vi "TakeAction.vi"(0 "Account Info":T1, 5 "Action":string, 7 "User input":string, 9 "Array":refnum<vi>[](array[refnum]), 11 "Error in":errorcluster) -> (4 "Get Message":string, 6 "Left menu":cluster{"L1":string, "L2":string, "L3":string}, 8 "Right Menu":cluster{"R1":string, "R2":string, "R3":string}, 10 "Updated acc info":T1, 15 "Error out":errorcluster)   [LabVIEW 2017]
doc: "This VI takes the appropriate action based on the action performed on the front panel. It also provides the output based on the action"
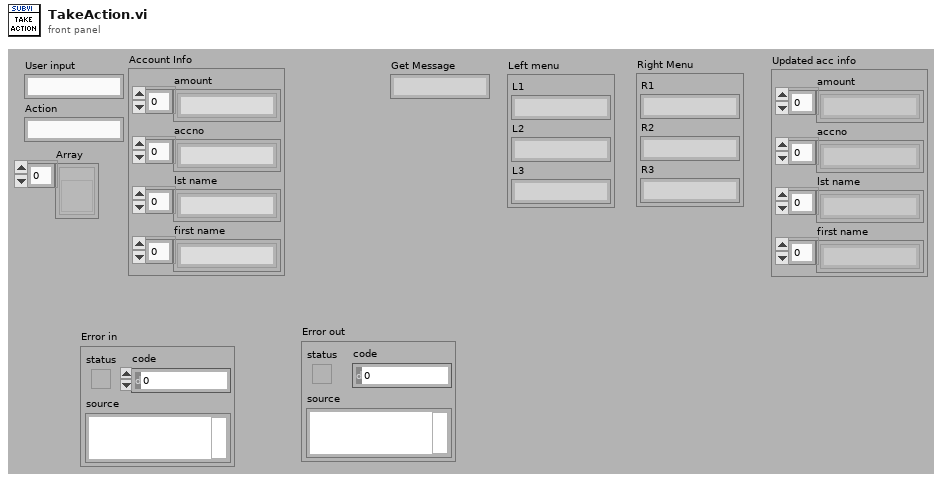
[diagram p1: front panel]
types:
  T1 = cluster{"amount":string[], "accno":string[], "lst name":string[], "first name":string[]}
  T2 = enum8{"Enabled", "Disabled", "Disabled and Grayed Out"}
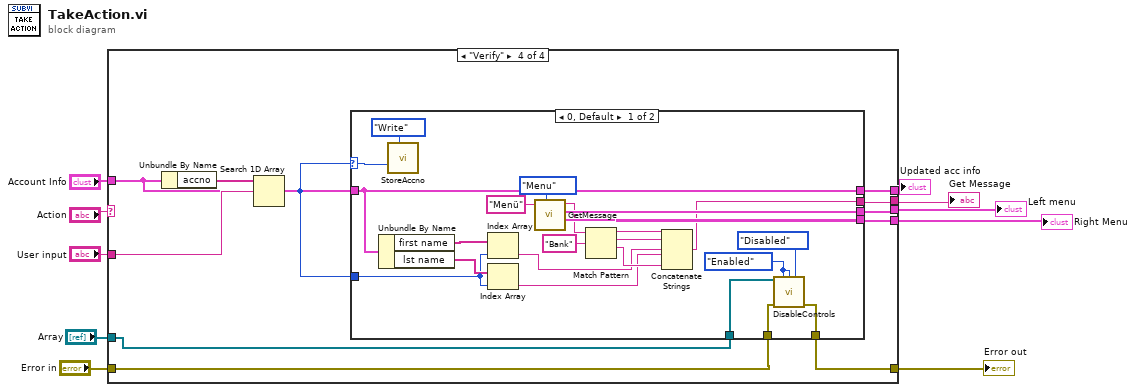
[diagram p0: block diagram]
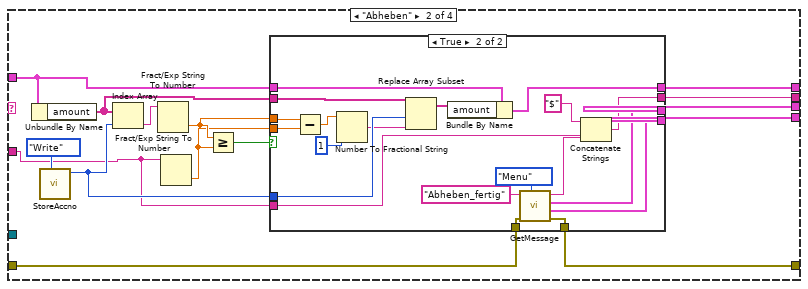
[diagram p3: hidden frame]
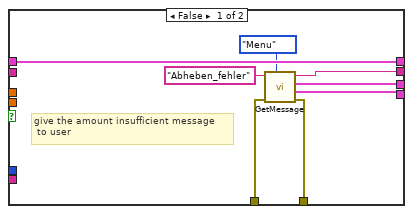
[diagram p4: hidden frame]
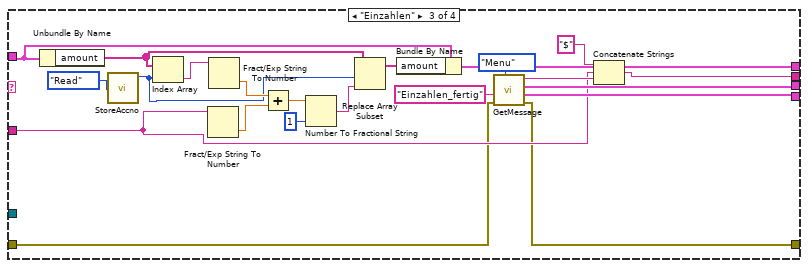
[diagram p5: hidden frame]
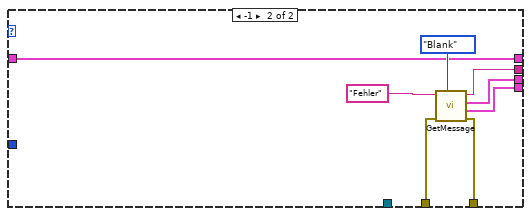
[diagram p6: hidden frame]
diagram:
  n1 = case shown="\"Verify\"" "Action" {
    tunnel: "User input" -> [_ w15 w58 w87]
    tunnel: "Account Info" -> [w12 w20 w73 w83]
    tunnel: [_ w16 w60 w86] -> w7
    tunnel: [_ w18 w66 w85] -> w6
    tunnel: [_ w17 w65 w84] -> w5
    tunnel: [w12 w19 w68 w82] -> w4
    tunnel: "Array" -> [_ _ _ w80]
    tunnel: "Error in" -> [w11 w14 w57 w79]
    tunnel: [w11 w13 w56 w78] -> w1
    frame Default {
    }
    frame "Abheben" {
      n2 = Unbundle By Name(w20) -> ("amount"=w21:string[])
      n3 = call "StoreAccno.vi"("Enum"=enum16{"Read", "Write"}."Write") -> ("Read"=w22:i32)  [unwired: 10 in]
      n4 = Index Array(array=w21, index=w22) -> (element=w26:string)
      n5 = Fract/Exp String To Number(string=w26) -> (number=w24:dbl)  [unwired: 3 in, 1 out]
      n6 = Fract/Exp String To Number(string=w15) -> (number=w23:dbl)  [unwired: 3 in, 1 out]
      n7 = Greater Or Equal?(x=w24, y=w23) -> (x >= y?=w25:bool)
      n8 = case shown="True" w25 {
        tunnel: w24 -> [_ w55]
        tunnel: w23 -> [_ w54]
        tunnel: w20 -> [w35 w53]
        tunnel: w22 -> [_ w50]
        tunnel: w21 -> [_ w52]
        tunnel: [w35 w48] -> w19
        tunnel: [w33 w41] -> w16
        tunnel: [w32 w46] -> w18
        tunnel: [w31 w45] -> w17
        tunnel: w15 -> [_ w39]
        tunnel: w14 -> [w29 w37]
        tunnel: [w28 w36] -> w13
        frame False {
          # "give the amount insufficient message\n to user"
          n9 = call "GetMessage.vi"("Action"=enum16{"Blank", "Menu"}."Menu", "Error in"=w29, "Message Type"="Abheben_fehler") -> ("Error Out"=w28:errorcluster, "Right Menu"=w31:cluster{"R1":string, "R2":string, "R3":string}, "Left menu"=w32:cluster{"L1":string, "L2":string, "L3":string}, "Get Message"=w33:string)  [unwired: 5 in]
        }
        frame True {
          n10 = Subtract(x=w55, y=w54) -> (x-y=w51:dbl)
          n11 = Number To Fractional String(number=w51, precision (6)=i16 1) -> (F-format string=w38:string)  [unwired: 2 in]
          n12 = Replace Array Subset(array=w52, new element=w38, index=w50) -> (w49:string[])
          n13 = Bundle By Name(cluster=w53, "amount"=w49) -> (w48:T1)
          n14 = call "GetMessage.vi"("Action"=enum16{"Blank", "Menu"}."Menu", "Error in"=w37, "Message Type"="Abheben_fertig") -> ("Error Out"=w36:errorcluster, "Right Menu"=w45:cluster{"R1":string, "R2":string, "R3":string}, "Left menu"=w46:cluster{"L1":string, "L2":string, "L3":string}, "Get Message"=w42:string)  [unwired: 5 in]
          n15 = Concatenate Strings("$" ("string"), w39, w42) -> (w41:string)
        }
      }
    }
    frame "Einzahlen" {
      n16 = Unbundle By Name(w73) -> ("amount"=w72:string[])
      n17 = call "StoreAccno.vi"("Enum"=enum16{"Read", "Write"}."Read") -> ("Read"=w71:i32)  [unwired: 10 in]
      n18 = Index Array(array=w72, index=w71) -> (element=w76:string)
      n19 = Fract/Exp String To Number(string=w58) -> (number=w74:dbl)  [unwired: 3 in, 1 out]
      n20 = Fract/Exp String To Number(string=w76) -> (number=w75:dbl)  [unwired: 3 in, 1 out]
      n21 = Add(x=w75, y=w74) -> (x+y=w70:dbl)
      n22 = Number To Fractional String(number=w70, precision (6)=i16 1) -> (F-format string=w62:string)  [unwired: 2 in]
      n23 = Replace Array Subset(array=w72, new element=w62, index=w71) -> (w69:string[])
      n24 = Bundle By Name(cluster=w73, "amount"=w69) -> (w68:T1)
      n25 = call "GetMessage.vi"("Action"=enum16{"Blank", "Menu"}."Menu", "Error in"=w57, "Message Type"="Einzahlen_fertig") -> ("Error Out"=w56:errorcluster, "Right Menu"=w65:cluster{"R1":string, "R2":string, "R3":string}, "Left menu"=w66:cluster{"L1":string, "L2":string, "L3":string}, "Get Message"=w61:string)  [unwired: 5 in]
      n26 = Concatenate Strings("$" ("string"), w58, w61) -> (w60:string)
    }
    frame "Verify" {
      n27 = Unbundle By Name(w83) -> ("accno"=w88:string[])
      n28 = Search 1D Array(1D array=w88, element=w87) -> (index of element=w81:i32)  [unwired: 1 in]
      n29 = case shown="0, Default" w81 {
        selector: w81 -> [w107 _]
        tunnel: [w101 w117] -> w86
        tunnel: [w110 w116] -> w85
        tunnel: [w109 w115] -> w84
        tunnel: w83 -> [w103 w114]
        tunnel: [w103 w114] -> w82
        tunnel: w81 -> [w102 _]
        tunnel: w80 -> [w96 _]
        tunnel: w79 -> [w93 w113]
        tunnel: [w92 w112] -> w78
        frame 0, Default {
          w95 = T2."Enabled" ("User Input")
          n30 = Unbundle By Name(w103) -> ("first name"=w105:string[], "lst name"=w104:string[])
          n31 = call "StoreAccno.vi"("Enum"=enum16{"Read", "Write"}."Write", "Numeric"=w107) -> ()  [unwired: 9 in, 1 out]
          n32 = Index Array(array=w105, index=w102) -> (element=w90:string)
          n33 = Index Array(array=w104, index=w102) -> (element=w89:string)
          n34 = call "GetMessage.vi"("Action"=enum16{"Blank", "Menu"}."Menu", "Message Type"="Menü") -> ("Right Menu"=w109:cluster{"R1":string, "R2":string, "R3":string}, "Left menu"=w110:cluster{"L1":string, "L2":string, "L3":string}, "Get Message"=w100:string)  [unwired: 6 in, 1 out]
          n35 = Match Pattern(string=w100, regular expression="Bank") -> (before substring=w98:string, match substring=w91:string, after substring=w97:string)  [unwired: 1 in, 1 out]
          n36 = Concatenate Strings(w98, w91, w90, w89, w97) -> (w101:string)
          n37 = call "DisableControls.vi"("Array"=w96, "User Input"=w95, "Menu action"=w95, "Card Simulator"=T2."Disabled", "Error In"=w93) -> ("Error Out"=w92:errorcluster)  [unwired: 10 in]
        }
        frame -1 {
          n38 = call "GetMessage.vi"("Action"=enum16{"Blank", "Menu"}."Blank", "Error in"=w113, "Message Type"="Fehler") -> ("Error Out"=w112:errorcluster, "Right Menu"=w115:cluster{"R1":string, "R2":string, "R3":string}, "Left menu"=w116:cluster{"L1":string, "L2":string, "L3":string}, "Get Message"=w117:string)  [unwired: 5 in]
        }
      }
    }
  }
  "Get Message" <- w7
  "Left menu" <- w6
  "Right Menu" <- w5
  "Error out" <- w1
  "Updated acc info" <- w4
